vi "Check Multiple Instances.vi"(8 "error in (no error)":errorcluster, 11 "Plugin in":refnum<class "Sift TDMS Uploader.lvclass">) -> (0 "error out":errorcluster, 3 "Plugin out":refnum<class "Sift TDMS Uploader.lvclass">)   [LabVIEW 2024, in "Sift TDMS Uploader.lvlib" / "Sift TDMS Uploader.lvclass"]
uses:
  Sift TDMS Uploader.lvclass
  C:/Program Files/National Instruments/LabVIEW 2024/vi.lib/FlexLogger/SDK/PluginSDK.lvlibp/PEFClasses/SDK/Processing Element/Processing Element.lvclass
  <vilib>/FlexLogger/SDK/PluginSDK.lvlibp/PEFClasses/SDK/Processing Element/Read System Interface.vi
  <vilib>/FlexLogger/SDK/PluginSDK.lvlibp/PEFClasses/SDK/Processing Element/Read Alias.vi
  Globals.vi
  <vilib>/FlexLogger/SDK/PluginSDK.lvlibp/PEFClasses/SDK/System Interface/System Interface.lvclass
  Sift TDMS Uploader.lvclass/Sift TDMS Uploader.ctl
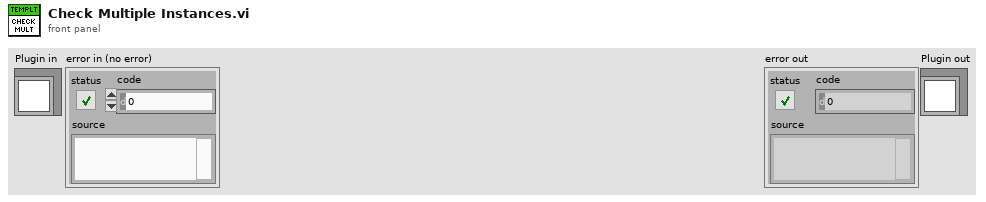
[diagram p1: front panel]
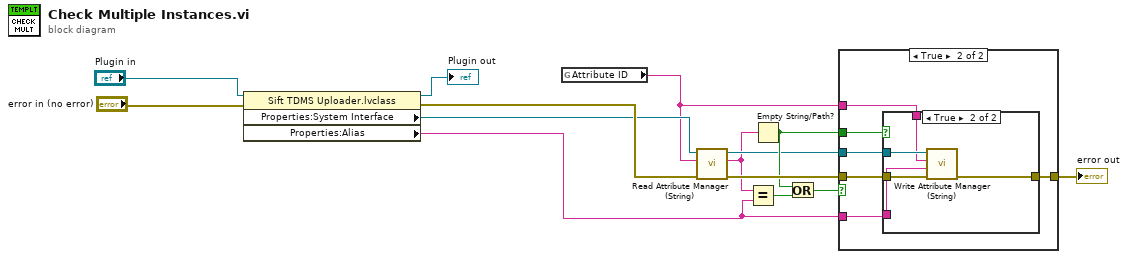
[diagram p0: block diagram]
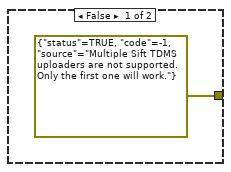
[diagram p2: hidden frame]
diagram:
  n1 = property class="Sift TDMS Uploader.lvclass"(reference="Plugin in", error in="error in (no error)") -> (reference out=→"Plugin out":refnum<class "Sift TDMS Uploader.lvclass">, error out=w7:errorcluster, "Properties:System Interface"=w4:refnum<class "System Interface.lvclass">, "Properties:Alias"=w3:string)
  n2 = global read "Globals.vi" "Attribute ID"() -> (w2:string)
  n3 = call-dynamic "Read Attribute Manager (String).vi"("error in (no error)"=w7, "Attribute ID"=w2, "System Interface in"=w4) -> ("error out"=w12:errorcluster, "Attrib Val"=w1:string, "System Interface out"=w9:refnum<class "System Interface.lvclass">)  [unwired: 5 in, 1 out]
  n4 = Equal?(x=w1, y=w3) -> (x = y?=w14:bool)
  n5 = Empty String/Path?(string/path=w1) -> (empty?=w10:bool)
  n6 = Or(x=w10, y=w14) -> (x .or. y?=w13:bool)
  n7 = case shown="True" w13 {
    tunnel: w12 -> [_ w20]
    tunnel: [errorcluster {"status"=TRUE, "code"=-1, "source"="Multiple Sift TDMS uploaders are not supported. Only the first one will work."} ("f") w16] -> w11
    tunnel: w10 -> [_ w17]
    tunnel: w2 -> [_ w19]
    tunnel: w9 -> [_ w21]
    tunnel: w3 -> [_ w18]
    frame False {
    }
    frame True {
      n8 = case shown="True" w17 {
        tunnel: w21 -> [_ w27]
        tunnel: w20 -> [w22 w26]
        tunnel: w19 -> [_ w25]
        tunnel: w18 -> [_ w24]
        tunnel: [w22 w23] -> w16
        frame False {
        }
        frame True {
          n9 = call-dynamic "Write Attribute Manager (String).vi"("error in (no error)"=w26, "Attribute Value"=w24, "Attribute ID"=w25, "System Interface in"=w27) -> ("error out"=w23:errorcluster)  [unwired: 5 in, 2 out]
        }
      }
    }
  }
  "error out" <- w11
